vi "Watch_Queue.vi"(8 "error in (no error)":errorcluster, 11 "QuWire in":refnum<class "QuWire.lvclass">) -> (0 "error out":errorcluster, 2 "Watch List":refnum<queue>, 3 "QuWire out":refnum<class "QuWire.lvclass">)   [LabVIEW 2020, in "QuWire.lvclass"]
uses:
  QuWire.lvclass
  QuWire.lvclass/QuWire.ctl
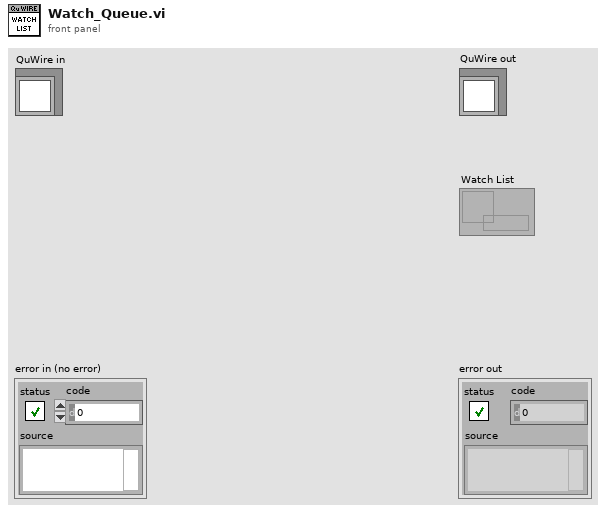
[diagram p1: front panel]
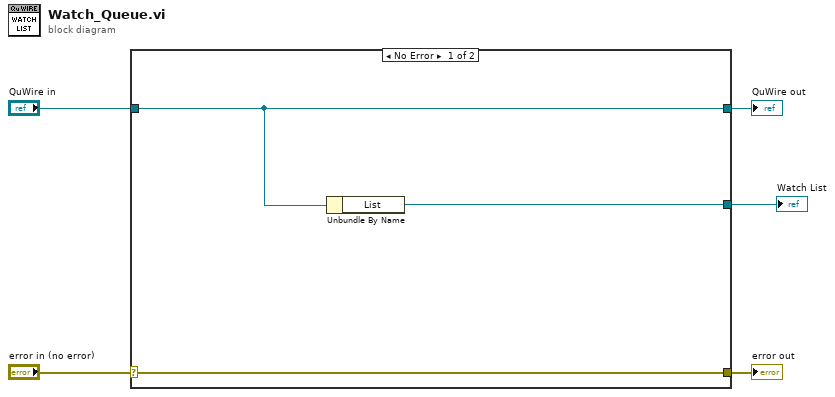
[diagram p0: block diagram]
diagram:
  n1 = case shown="No Error" "error in (no error)" {
    selector: "error in (no error)" -> [w8 w10]
    tunnel: [w8 w10] -> w4
    tunnel: [w7 w9] -> w2
    tunnel: "QuWire in" -> [w7 w9]
    tunnel: [w6 _] -> w1
    frame No Error {
      n2 = Unbundle By Name(w7) -> ("List"=w6:refnum<queue>)
    }
    frame Error {
    }
  }
  "error out" <- w4
  "QuWire out" <- w2
  "Watch List" <- w1
